vi "TicTacToe.vi"() -> ()   [LabVIEW 2017]
uses:
  Opponent.vi
panel:
  in  "Smart Computer":bool
  in  "New Game":bool
  in  "New Round":bool
  out "Score 2":i32
  out "Score 1":i32
  out "Status":string
  in  "Matrix":T1
  in  "Player 2":bool
  in  "Player 1":bool=TRUE
  # "Score"
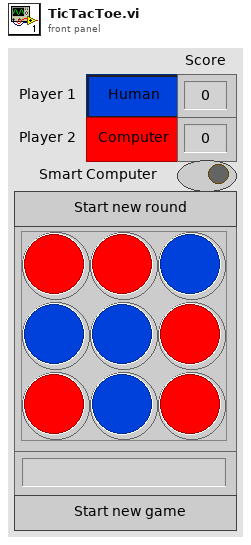
[diagram p1: front panel]
types:
  T1 = cluster{"0":bool, "1":bool, "2":bool, "3":bool, "4":bool, "5":bool, "6":bool, "7":bool, "8":bool}
  T2 = enum8{"Enabled", "Disabled", "Disabled and Grayed Out"}
  T3 = cluster{"Tokens":i32[][], "Score 1":i32, "Score 2":i32, "CurrentPlayer":i32, "FrontPanel":refnum<vi>, "StartPlayer":i32, "RoundRunning":bool}
  T4 = cluster{"Matrix[0]":bool, "Matrix[1]":bool, "Matrix[2]":bool, "Matrix[3]":bool, "Matrix[4]":bool, "Matrix[5]":bool, "Matrix[6]":bool, "Matrix[7]":bool, "Matrix[8]":bool}
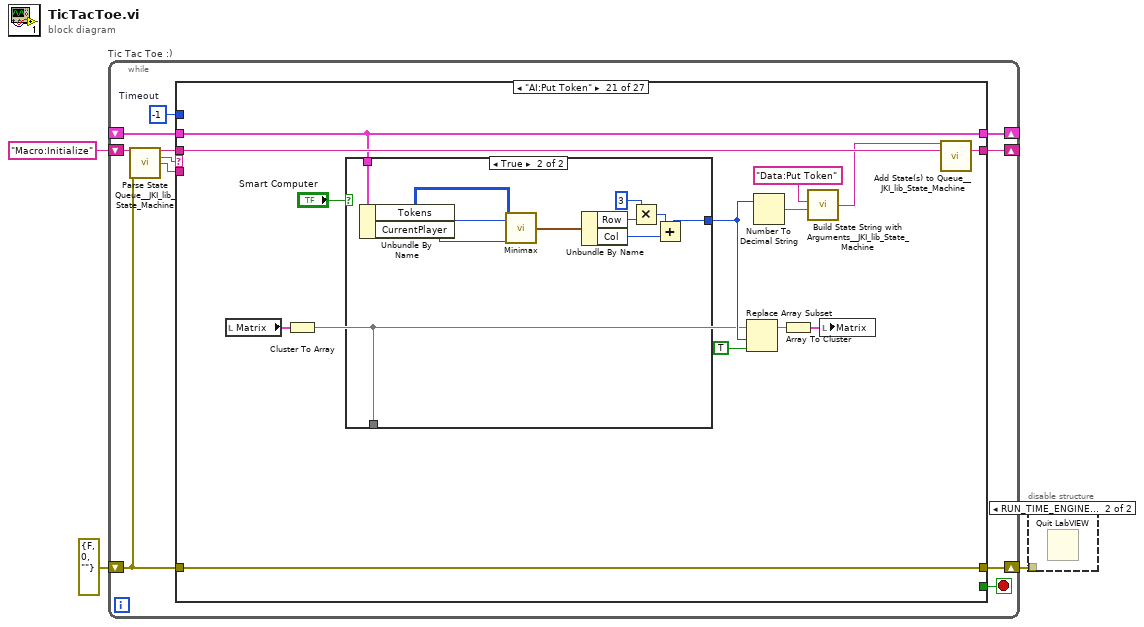
[diagram p0: block diagram]
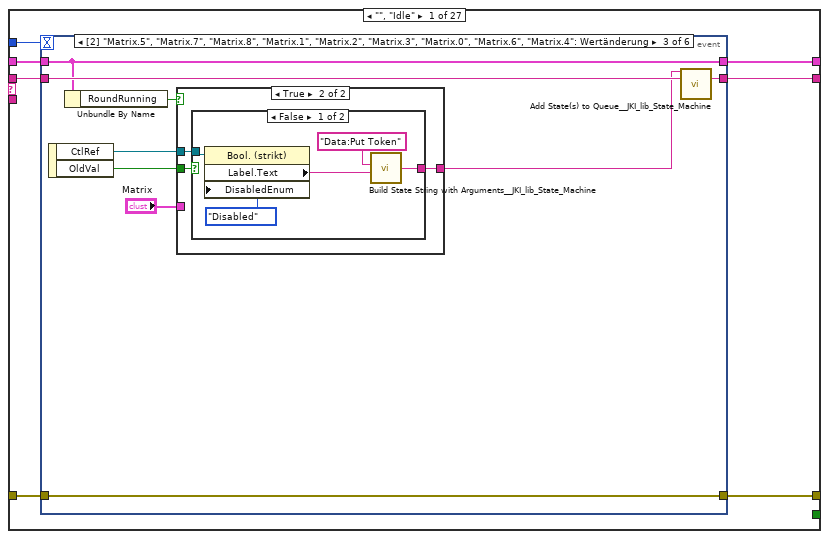
[diagram p3: hidden frame]
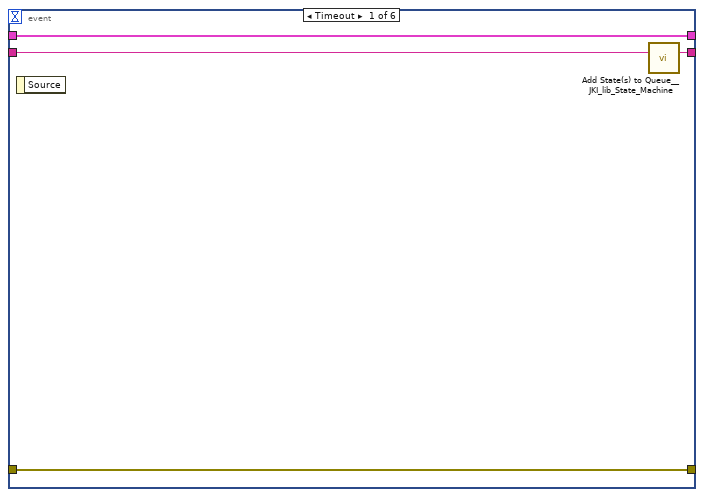
[diagram p4: hidden frame]
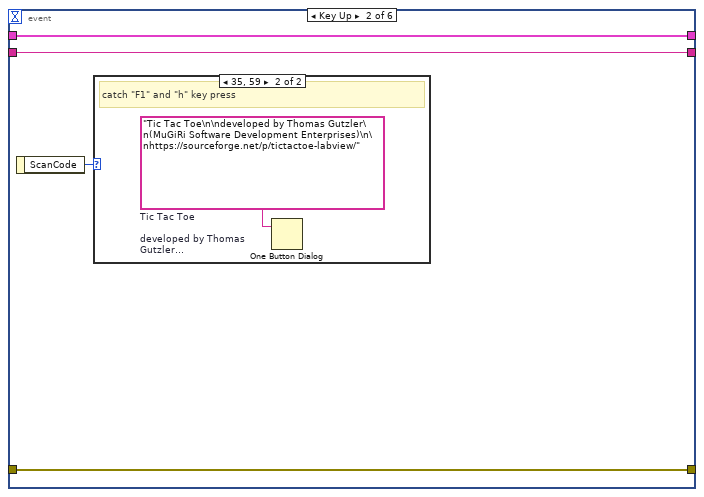
[diagram p5: hidden frame]
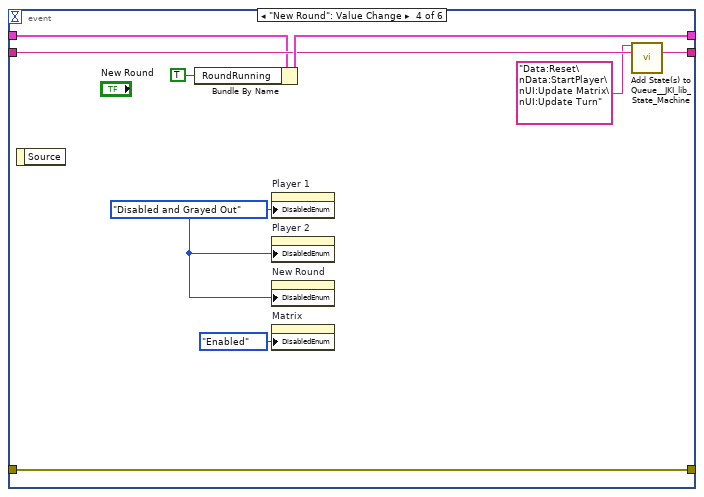
[diagram p9: hidden frame]
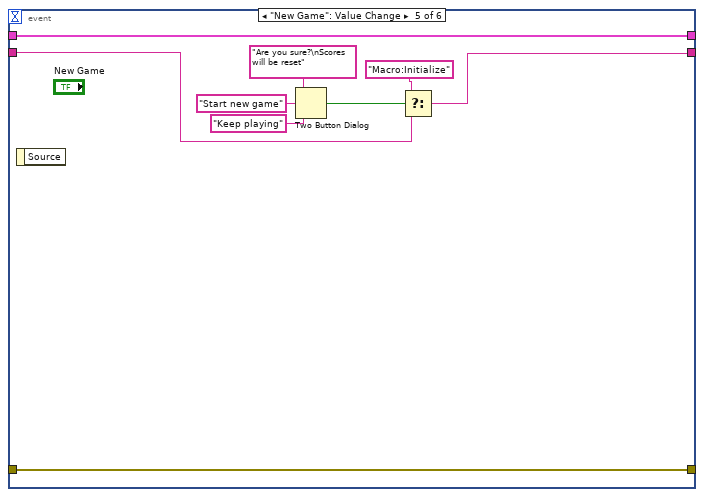
[diagram p10: hidden frame]
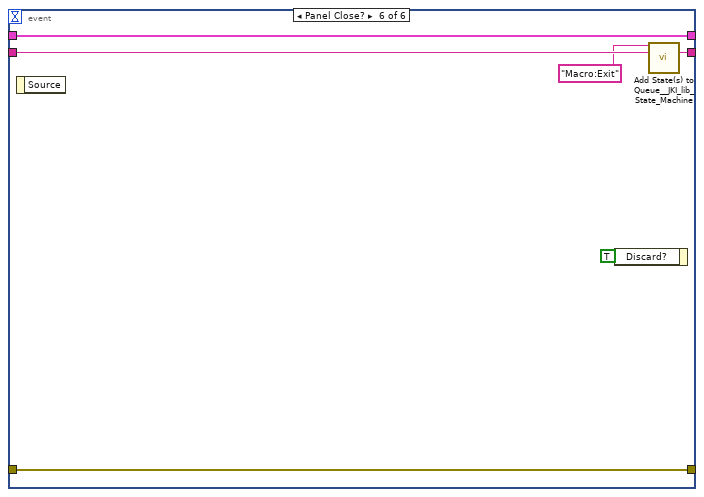
[diagram p11: hidden frame]
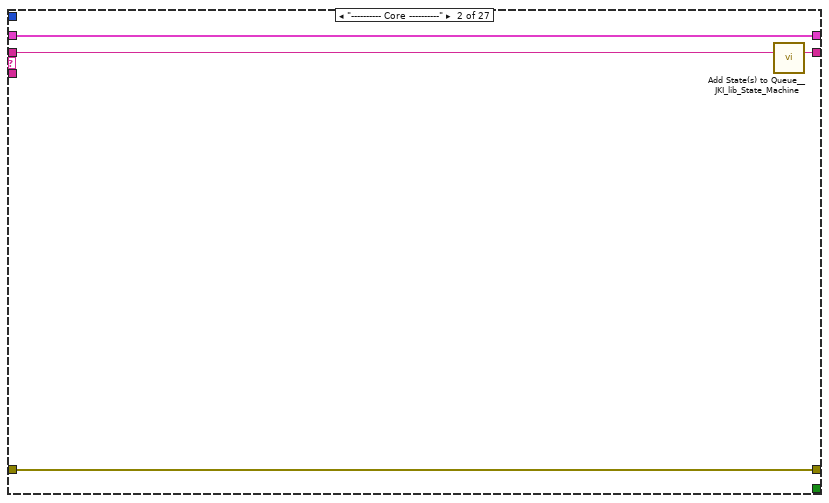
[diagram p12: hidden frame]
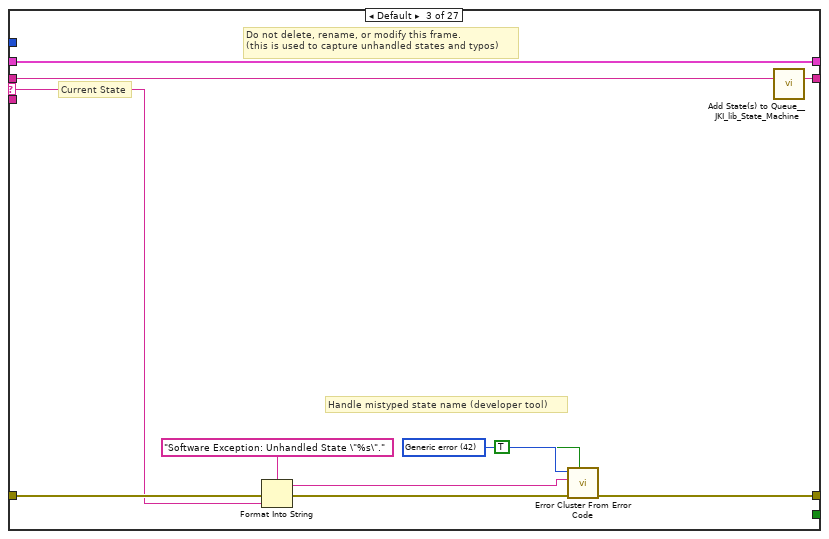
[diagram p13: hidden frame]
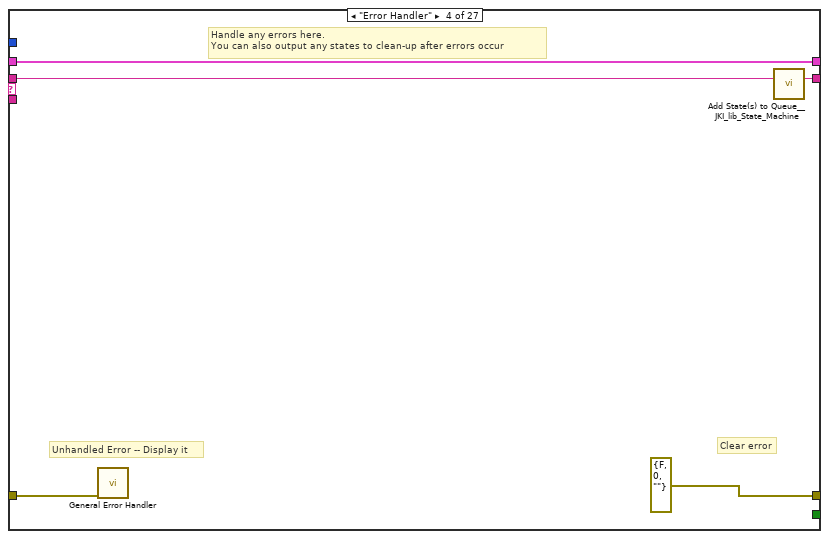
[diagram p14: hidden frame]
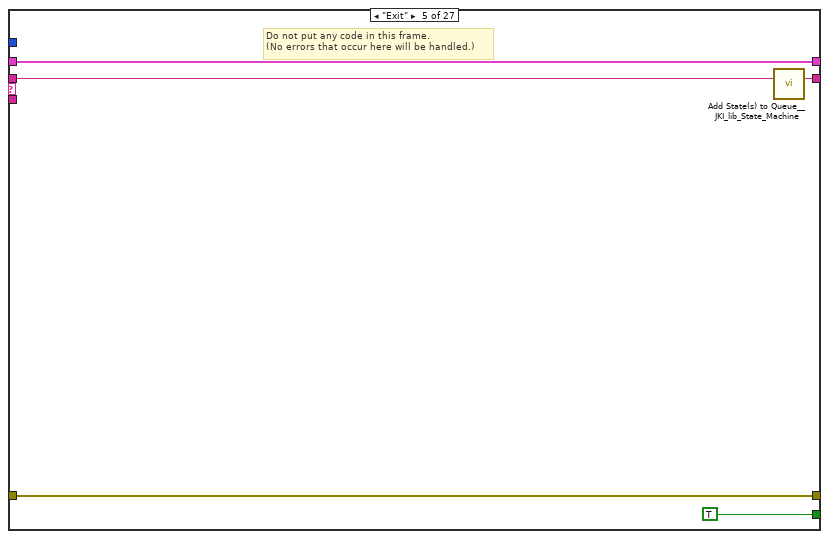
[diagram p15: hidden frame]
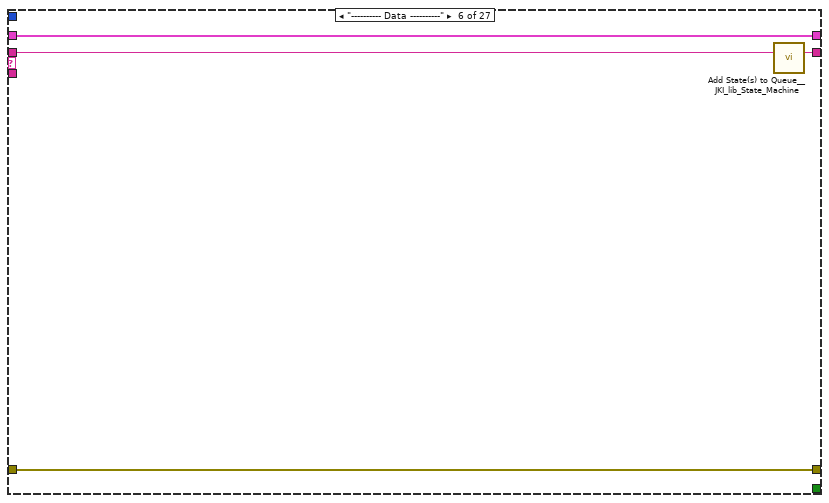
[diagram p16: hidden frame]
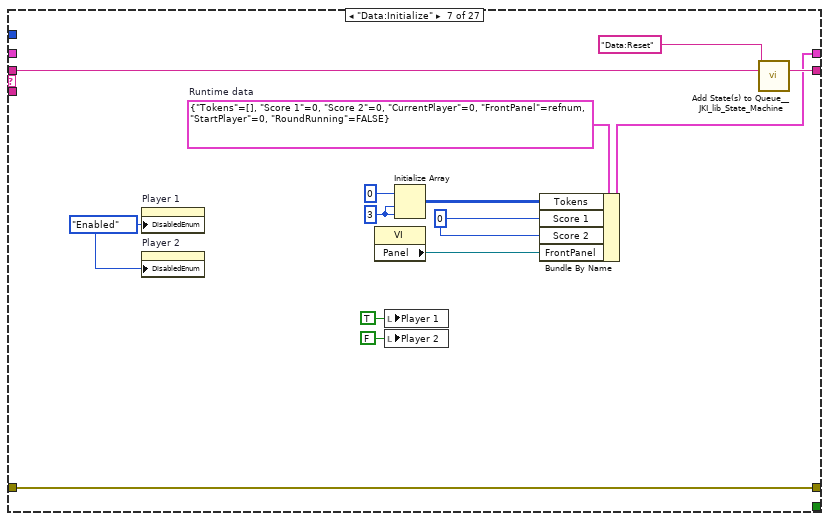
[diagram p17: hidden frame]
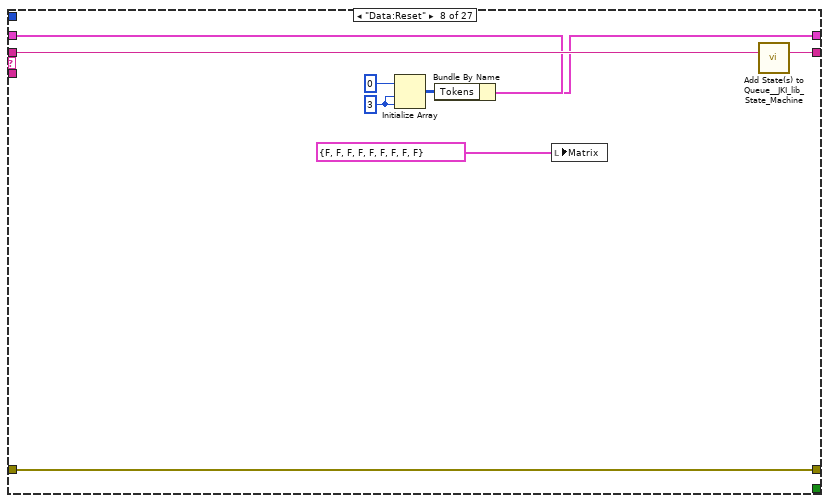
[diagram p18: hidden frame]
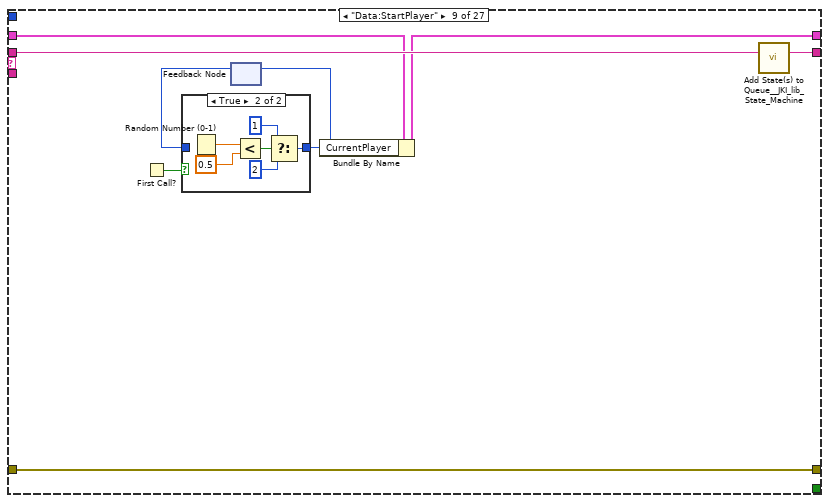
[diagram p19: hidden frame]
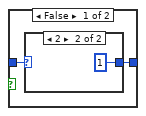
[diagram p20: hidden frame]
diagram:
  n1 = while "Tic Tac Toe :)" {
    shift-right: [w7] -> _
    shift-left: _ -> [w6]
    shift-right: [w10] -> w1
    shift-left: errorcluster {"status"=FALSE, "code"=0, "source"=""} ("error out") -> [w4]
    shift-right: [w9] -> _
    shift-left: "Macro:Initialize" -> [w11]
    stop <- w8 stop-if-true
    w5 = -1  # Timeout
    n2 = call <vilib>:"Parse State Queue__JKI_lib_State_Machine.vi"("State Queue"=w11, "Error In (no error)"=w4) -> ("Remaining States"=w13:string, "Current State"=w14:string, "Arguments"=w12:string)  [unwired: 11 in]
    n3 = case shown="\"AI:Put Token\"" w14 {
      selector: w14 -> [_ _ w76 _ _ _ _ _ _ _ _ _ _ _ _ _ _ _ _ _ _ _ _ _ _ _ _]
      tunnel: w13 -> [w21 w75 w80 w91 w96 w100 w114 w123 w131 w144 w180 w184 w193 w207 w230 w237 w242 w248 w252 w265 w279 w303 w308 w313 w317 _ _]
      tunnel: w12 -> [_ _ _ _ _ _ _ _ _ w162 w174 _ _ _ _ _ w239 _ _ _ _ _ _ _ _ w320 _]
      tunnel: w6 -> [w19 w72 w78 w88 w94 w97 _ w117 w128 w155 w177 w181 w191 w203 w227 w232 w240 w246 w249 w262 w269 w300 w305 w310 w314 w326 w342]
      tunnel: [w18 w73 w82 errorcluster {"status"=FALSE, "code"=0, "source"=""} ("error out") w93 w98 w112 w121 w129 w163 w178 w182 w190 w205 w228 w235 w238 w245 w250 w263 w277 w301 w306 w311 w315 w329 w348] -> w10
      tunnel: w4 -> [w17 w73 w81 w87 w93 w98 w112 w121 w129 w163 w178 w182 w190 w205 w228 w235 w238 w245 w250 w263 w277 w301 w306 w311 w315 w329 w348]
      tunnel: [w20 w74 w79 w90 w95 w99 w113 w122 w130 w145 w179 w183 w192 w206 w229 w236 w241 w247 w251 w264 w278 w302 w307 w312 w316 w330 "UI:Status >> Game Over"] -> w9
      tunnel: [_ _ _ _ TRUE _ _ _ _ _ _ _ _ _ _ _ _ _ _ _ _ _ _ _ _ _ _] -> w8
      tunnel: [w16 w72 w78 w88 w94 w97 w110 w116 w127 w160 w177 w181 w191 w203 w227 w232 w240 w246 w249 w262 w269 w300 w305 w310 w314 w325 w341] -> w7
      tunnel: w5 -> [w15 _ _ _ _ _ _ _ _ _ _ _ _ _ _ _ _ _ _ _ _ _ _ _ _ _ _]
      frame "", "Idle" {
        n4 = event shown="[2] \"Matrix.5\", \"Matrix.7\", \"Matrix.8\", \"Matrix.1\", \"Matrix.2\", \"Matrix.3\", \"Matrix.0\", \"Matrix.6\", \"Matrix.4\": Wertänderung" {
          selector: _ -> [_ _ _ _ _ _]
          dyn-events: _ -> [_ _ _ _ _ _]
          timeout: w15 -> [_ _ _ _ _ _]
          tunnel: w21 -> [w25 w27 w39 w53 w59 w71]
          tunnel: [w24 w27 w38 w52 w58 w70] -> w20
          tunnel: w19 -> [w22 w28 w31 w50 w65 w68]
          tunnel: [w23 w29 w37 w56 w57 w69] -> w18
          tunnel: w17 -> [w23 w29 w37 w56 w57 w69]
          tunnel: [w22 w28 w31 w55 w65 w68] -> w16
          event Timeout {
            n5 = event-data() -> ()  [unwired: 1 in, 1 out]
            n6 = call <vilib>:"Add State(s) to Queue__JKI_lib_State_Machine.vi"("State(s) in (\"\")"=w25) -> ("States Out"=w24:string)  [unwired: 14 in]
          }
          event Key Up {
            n7 = event-data() -> ("ScanCode"=w26:i16)  [unwired: 1 in]
            n8 = case shown="35, 59" w26 {
              frame 0, Default {
              }
              frame 35, 59 {
                w30 = "Tic Tac Toe\n\ndeveloped by Thomas Gutzler\n(MuGiRi Software Development Enterprises)\n\nhttps://sourceforge.net/p/tictactoe-labview/"  # Tic Tac Toe  developed by Thomas Gutzler (MuGiRi Software Development Enterprises)  https://sourceforge.net/p/tictactoe-labview/
                # "catch \"F1\" and \"h\" key press"
                n9 = One Button Dialog(message=w30) -> ()  [unwired: 1 in, 1 out]
              }
            }
          }
          event "Matrix.5", "Matrix.7", "Matrix.8", "Matrix.1", "Matrix.2", "Matrix.3", "Matrix.0", "Matrix.6", "Matrix.4": Value Change {
            n10 = event-data() -> ("CtlRef"=w36:refnum<vi>, "OldVal"=w34:bool)  [unwired: 1 in]
            n11 = Unbundle By Name(w31) -> ("RoundRunning"=w33:bool)
            n12 = case shown="True" w33 {
              tunnel: w36 -> [_ w42]
              tunnel: [_ w41] -> w35
              tunnel: w34 -> [_ w40]
              tunnel: "Matrix" -> [_ _]
              frame False {
              }
              frame True {
                n13 = case shown="False" w40 {
                  tunnel: w42 -> [w47 _]
                  tunnel: [w44 _] -> w41
                  frame False {
                    n14 = property class="Bool. (strikt)"(reference=w47, "DisabledEnum"=T2."Disabled" ("Disabled")) -> ("Label.Text"=w45:string)  [unwired: 1 in, 2 out]
                    n15 = call <vilib>:"Build State String with Arguments__JKI_lib_State_Machine.vi"("Arguments (\"\")"=w45, "State"="Data:Put Token") -> ("State with Arguments"=w44:string)  [unwired: 4 in]
                  }
                  frame True {
                  }
                }
              }
            }
            n16 = call <vilib>:"Add State(s) to Queue__JKI_lib_State_Machine.vi"("State(s) in Front (\"\")"=w35, "State(s) in (\"\")"=w39) -> ("States Out"=w38:string)  [unwired: 13 in]
          }
          event "New Round": Value Change {
            w51 = T2."Disabled and Grayed Out" ("Disabled")
            n17 = event-data() -> ()  [unwired: 1 in, 1 out]
            n18 = Bundle By Name(cluster=w50, "RoundRunning"=TRUE ("GameRunning")) -> (w55:T3)
            n19 = property on="Player 1" class="Bool. (strikt)"("DisabledEnum"=w51) -> ()  [unwired: 2 in, 2 out]
            n20 = property on="Player 2" class="Bool. (strikt)"("DisabledEnum"=w51) -> ()  [unwired: 2 in, 2 out]
            n21 = property on="New Round" class="Bool. (strikt)"("DisabledEnum"=w51) -> ()  [unwired: 2 in, 2 out]
            n22 = property on="Matrix" class="Cluster (strikt)"("DisabledEnum"=T2."Enabled" ("Disabled")) -> ()  [unwired: 2 in, 2 out]
            n23 = call <vilib>:"Add State(s) to Queue__JKI_lib_State_Machine.vi"("State(s) in Front (\"\")"="Data:Reset\nData:StartPlayer\nUI:Update Matrix\nUI:Update Turn", "State(s) in (\"\")"=w53) -> ("States Out"=w52:string)  [unwired: 13 in]
          }
          event "New Game": Value Change {
            n24 = event-data() -> ()  [unwired: 1 in, 1 out]
            n25 = Two Button Dialog(message="Are you sure?\nScores will be reset", 1:"Keep playing", 2:"Start new game" ("T button name (\"OK\")")) -> (T button?=w61:bool)
            n26 = Select(t="Macro:Initialize", s=w61, f=w59) -> (s? t:f=w58:string)
          }
          event Panel Close? {
            n27 = event-data() -> ()  [unwired: 1 in, 1 out]
            n28 = event-data("Discard?"=TRUE) -> ()  [unwired: 1 in, 1 out]
            n29 = call <vilib>:"Add State(s) to Queue__JKI_lib_State_Machine.vi"("State(s) in Front (\"\")"="Macro:Exit", "State(s) in (\"\")"=w71) -> ("States Out"=w70:string)  [unwired: 13 in]
          }
        }
      }
      frame "---------- Core ----------" {
        n30 = call <vilib>:"Add State(s) to Queue__JKI_lib_State_Machine.vi"("State(s) in (\"\")"=w75) -> ("States Out"=w74:string)  [unwired: 14 in]
      }
      frame Default {
        w85 = 42 items=["No error", "Argument error", "Memory is full", "Out of zone", "End of file", "File already open", "Generic file I/O error", "File not found", "File permission error", "Disk is full", "Duplicate path", "Too many files open", "System feature not enabled", "Resource file not found", "Cannot add resource", "Resource not found", "Image not found", "Image memory error", "Pen does not exist", "Config type invalid", "Config token not found", "Config parse error", "Config memory error", "Bad external code format", "Bad external code offset", "External code not present", "Null window", "Destroy window error", "Null menu", "Print aborted", "Bad print record", "Print driver error", "Windows error during printing", "Memory error during printing", "Print dialog error", "Generic print error", "Invalid device refnum", "Device not found", "Device parameter error", "Device unit error", "Cannot open device", "Device call aborted", "Generic error", "Cancelled by user", "Object ID too low", "Object ID too high", "Object not in heap", "Unknown heap", "Unknown object (invalid DefProc)", "Unknown object (DefProc not in table)", "Message out of range", "Invalid (null) method", "Unknown message", "Manager call not supported", "Bad address", "Network operation in progress", "Network operation timed out", "Connection is busy", "Network attribute not supported", "Network error", "Address in use", "System out of memory", "Connection aborted", "Connection refused", "Not connected", "Already connected", "Connection closed", "Initialization error (interapplication manager)", "Bad occurrence", "Wait on unbound occurrence handler", "Occurrence queue overflow", "Datalog type conflict", "Unused", "Unrecognized type (interapplication manager)", "Memory corrupt", "Failed to make temporary DLL", "Old CIN version", "Drag socket not found", "Failed to load drop-object", "Failed to register OLE object", "Failed to release OLE object", "Format specifier type mismatch", "Unknown format specifier", "Too few format specifiers", "Too many format specifiers", "Scan failed", "Newer CIN version", "Error converting to variant", "Runtime menu error", "Password tampered", "Variant attribute not found", "Incompatible variant data type", "Event data is not available", "Event Store is not present", "Occurrence is not found", "Event Queue is not created", "Event info is not available", "Refnum passed is NULL", "Error retrieving Class GUID", "Error retrieving CoClass GUID", "Error retrieving TypeLib GUID.", "Bad built application magic bytes.", "Specific driver is different from the specific driver associated with the Logical Name.", "There is no session opened to the class driver.", "Max Error", "MAX - Error with config objects", "MAX - Error loading configuration", "MAX - Group not supported"]
        # "Current State"
        # "Do not delete, rename, or modify this frame.\n(this is used to capture unhandled states and typos)"
        # "Handle mistyped state name (developer tool)"
        n31 = Format Into String(format string="Software Exception: Unhandled State \"%s\"." ("message"), error in=w81, w76) -> (resulting string=w84:string, error out=w83:errorcluster)  [unwired: 1 in]
        n32 = call <vilib>:"Error Cluster From Error Code.vi"("show call chain? (False)"=TRUE, "error in (no error)"=w83, "error message (\"\")"=w84, "error code (0)"=w85) -> ("error out"=w82:errorcluster)  [unwired: 5 in]
        n33 = call <vilib>:"Add State(s) to Queue__JKI_lib_State_Machine.vi"("State(s) in (\"\")"=w80) -> ("States Out"=w79:string)  [unwired: 14 in]
      }
      frame "Error Handler" {
        # "Unhandled Error -- Display it"
        # "Handle any errors here.\nYou can also output any states to clean-up after errors occur"
        # "Clear error"
        n34 = call <vilib>:"General Error Handler.vi"("error in (no error)"=w87) -> ()  [unwired: 10 in, 5 out]
        n35 = call <vilib>:"Add State(s) to Queue__JKI_lib_State_Machine.vi"("State(s) in (\"\")"=w91) -> ("States Out"=w90:string)  [unwired: 14 in]
      }
      frame "Exit" {
        # "Do not put any code in this frame.\n(No errors that occur here will be handled.)"
        n36 = call <vilib>:"Add State(s) to Queue__JKI_lib_State_Machine.vi"("State(s) in (\"\")"=w96) -> ("States Out"=w95:string)  [unwired: 14 in]
      }
      frame "---------- Data ----------" {
        n37 = call <vilib>:"Add State(s) to Queue__JKI_lib_State_Machine.vi"("State(s) in (\"\")"=w100) -> ("States Out"=w99:string)  [unwired: 14 in]
      }
      frame "Data:Initialize" {
        w102 = T2."Enabled" ("Disabled")
        w105 = 3 ("Score 1")
        w107 = 0 ("Score 1")
        w111 = T3 {"Tokens"=[], "Score 1"=0, "Score 2"=0, "CurrentPlayer"=0, "FrontPanel"=refnum, "StartPlayer"=0, "RoundRunning"=FALSE}  # Runtime data
        n38 = property on="Player 1" class="Bool. (strikt)"("DisabledEnum"=w102) -> ()  [unwired: 2 in, 2 out]
        n39 = property on="Player 2" class="Bool. (strikt)"("DisabledEnum"=w102) -> ()  [unwired: 2 in, 2 out]
        n40 = property class="VI"() -> ("Panel"=w106:refnum<vi>)  [unwired: 2 in, 2 out]
        n41 = local write "Player 1"(TRUE ("Player 1")) -> ()
        n42 = local write "Player 2"(FALSE ("Player 2")) -> ()
        n43 = Initialize Array(0 ("Score 1"), w105, w105) -> (w108:i32[][])
        n44 = Bundle By Name(cluster=w111, "Tokens"=w108, "Score 1"=w107, "Score 2"=w107, "FrontPanel"=w106) -> (w110:T3)
        n45 = call <vilib>:"Add State(s) to Queue__JKI_lib_State_Machine.vi"("State(s) in Front (\"\")"="Data:Reset", "State(s) in (\"\")"=w114) -> ("States Out"=w113:string)  [unwired: 13 in]
      }
      frame "Data:Reset" {
        w118 = 3 ("Score 1")
        n46 = Initialize Array(0 ("Score 1"), w118, w118) -> (w119:i32[][])
        n47 = Bundle By Name(cluster=w117, "Tokens"=w119) -> (w116:T3)
        n48 = local write "Matrix"(T1 {"0"=FALSE, "1"=FALSE, "2"=FALSE, "3"=FALSE, "4"=FALSE, "5"=FALSE, "6"=FALSE, "7"=FALSE, "8"=FALSE} ("Matrix")) -> ()
        n49 = call <vilib>:"Add State(s) to Queue__JKI_lib_State_Machine.vi"("State(s) in (\"\")"=w123) -> ("States Out"=w122:string)  [unwired: 14 in]
      }
      frame "Data:StartPlayer" {
        n50 = First Call?() -> (First Call?: T/F=w126:bool)
        n51 = feedback #1() -> (w124:i32)  [unwired: 1 in]
        n52 = case shown="True" w126 {
          tunnel: [w132 w136] -> w125
          tunnel: w124 -> [w133 _]
          frame False {
            n53 = case shown="2" w133 {
              tunnel: [2 1] -> w132
              frame Default {
              }
              frame 2 {
              }
            }
          }
          frame True {
            n54 = Random Number (0-1)() -> (number: 0 to 1=w141:dbl)
            n55 = Less?(x=w141, y=0.5 ("x")) -> (x < y?=w139:bool)
            n56 = Select(t=1 ("Score 2"), s=w139, f=2 ("Score 2")) -> (s? t:f=w136:i32)
          }
        }
        n57 = feedback-in #1(w125) -> ()
        n58 = Bundle By Name(cluster=w128, "CurrentPlayer"=w125) -> (w127:T3)
        n59 = call <vilib>:"Add State(s) to Queue__JKI_lib_State_Machine.vi"("State(s) in (\"\")"=w131) -> ("States Out"=w130:string)  [unwired: 14 in]
      }
      frame "Data:Put Token" {
        w153 = 3 ("dimension size")
        n60 = Decimal String To Number(string=w162) -> (number=w161:i32)  [unwired: 2 in, 1 out]
        n61 = Unbundle By Name(w155) -> ("CurrentPlayer"=w149:i32)
        n62 = Unbundle By Name(w155) -> ("Tokens"=w157:i32[][])
        n63 = Reshape Array(w157, 9 ("dimension size")) -> (w156:i32[])
        n64 = Replace Array Subset(array=w156, new element=w149, index=w161) -> (w154:i32[])
        n65 = case shown="Standard" w149 {
          tunnel: [1 ("CurrentPlayer") 2 ("CurrentPlayer")] -> w151
          frame Default {
          }
          frame 1 {
          }
        }
        n66 = Number To Decimal String(number=w149) -> (decimal integer string=w148:string)  [unwired: 1 in]
        n67 = Reshape Array(w154, w153, w153) -> (w152:i32[][])
        n68 = Bundle By Name(cluster=w155, "Tokens"=w152, "CurrentPlayer"=w151) -> (w160:T3)
        n69 = call <vilib>:"Build State String with Arguments__JKI_lib_State_Machine.vi"("Arguments (\"\")"=w148, "State"="Data:Check Win") -> ("State with Arguments"=w147:string)  [unwired: 4 in]
        n70 = call <vilib>:"Add State(s) to Queue__JKI_lib_State_Machine.vi"("State(s) in Front (\"\")"="UI:Update Turn", "State(s) in (\"\")"=w144) -> ("States Out"=w143:string)  [unwired: 13 in]
        n71 = call <vilib>:"Add State(s) to Queue__JKI_lib_State_Machine.vi"("State(s) in Front (\"\")"=w147, "State(s) in (\"\")"=w143) -> ("States Out"=w146:string)  [unwired: 13 in]
        n72 = call <vilib>:"Add State(s) to Queue__JKI_lib_State_Machine.vi"("State(s) in Front (\"\")"="UI:Update Matrix", "State(s) in (\"\")"=w146) -> ("States Out"=w145:string)  [unwired: 13 in]
      }
      frame "Data:Check Win" {
        n73 = Unbundle By Name(w177) -> ("Tokens"=w172:i32[][])
        n74 = Decimal String To Number(string=w174) -> (number=w171:i32)  [unwired: 2 in, 1 out]
        n75 = call "Score.vi"("Turn Taking Player"=w171, "Game"=w172) -> ("Game over"=w169:bool, "Win"=w170:bool)  [unwired: 7 in, 1 out]
        n76 = Select(t="Game:Over", s=w169, f="") -> (s? t:f=w166:string)
        n77 = call <vilib>:"Build State String with Arguments__JKI_lib_State_Machine.vi"("Arguments (\"\")"=w174, "State"="Game:Winner") -> ("State with Arguments"=w173:string)  [unwired: 4 in]
        n78 = Select(t=w173, s=w170, f=w166) -> (s? t:f=w176:string)
        n79 = call <vilib>:"Add State(s) to Queue__JKI_lib_State_Machine.vi"("State(s) in Front (\"\")"=w176, "State(s) in (\"\")"=w180) -> ("States Out"=w179:string)  [unwired: 13 in]
      }
      frame "---------- UI ----------" {
        n80 = call <vilib>:"Add State(s) to Queue__JKI_lib_State_Machine.vi"("State(s) in (\"\")"=w184) -> ("States Out"=w183:string)  [unwired: 14 in]
      }
      frame "UI:Initialize" {
        # "Initialize the User Interface, here.\n(this is called automatically, by the Macro: Init)"
        n81 = property on="New Round" class="Bool. (strikt)"("DisabledEnum"=T2."Enabled" ("Disabled")) -> ()  [unwired: 2 in, 2 out]
        n82 = property on="Matrix" class="Cluster (strikt)"("DisabledEnum"=T2."Disabled" ("Disabled")) -> ()  [unwired: 2 in, 2 out]
        n83 = local write "New Round"(FALSE ("Start")) -> ()
        n84 = local write "Matrix"(T1 {"0"=FALSE, "1"=FALSE, "2"=FALSE, "3"=FALSE, "4"=FALSE, "5"=FALSE, "6"=FALSE, "7"=FALSE, "8"=FALSE} ("Matrix")) -> ()
        n85 = call <vilib>:"Add State(s) to Queue__JKI_lib_State_Machine.vi"("State(s) in Front (\"\")"="UI:Status\nUI:Update Score\nUI:Update Matrix", "State(s) in (\"\")"=w193) -> ("States Out"=w192:string)  [unwired: 13 in]
      }
      frame "UI:Update Matrix" {
        n86 = Unbundle By Name(w203) -> ("FrontPanel"=w202:refnum<vi>)
        n87 = property class="Pnl"(reference=w202, "DeferPanUpdts"=TRUE ("Defer Panel Updates")) -> (reference out=w199:refnum<vi>, error out=w200:errorcluster)  [unwired: 1 in]
        n88 = property on="Matrix" class="Cluster (strikt)"(error in=w200) -> ("Controls[]"=w204:refnum<vi>[])  [unwired: 1 in, 2 out]
        n89 = Unbundle By Name(w203) -> ("Tokens"=w196:i32[][])
        n90 = Reshape Array(w196, 9 ("dimension size")) -> (w194:i32[])
        n91 = for {
          tunnel: w204 -> [w218] mode=indexing
          tunnel: w194 -> [w212]
          tunnel: [w210] -> w198
          w216 = refnum<vi> refnum  # Boolesch
          n92 = To More Specific Class(target class=w216, reference=w218) -> (specific class reference=w217:refnum<vi>)  [unwired: 1 in, 1 out]
          n93 = property class="Bool."(reference=w217) -> (reference out=w215:refnum<vi>, "Label.Text"=w214:string)  [unwired: 1 in, 1 out]
          n94 = Decimal String To Number(string=w214) -> (number=w213:i32)  [unwired: 2 in, 1 out]
          n95 = Index Array(array=w212, index=w213) -> (element=w209:i32)
          n96 = case shown="Standard" w209 {
            tunnel: [cluster{u32, u32}[] [{13816530, 13816530}, {13816530, 13816530}] ("Colors [4]") cluster{u32, u32}[] [{16860, 16860}, {16860, 16860}] ("Colors [4]") cluster{u32, u32}[] [{16711680, 16711680}, {16711680, 16711680}] ("Colors [4]")] -> w211
            tunnel: [T2."Enabled" ("Disabled") T2."Disabled" ("Disabled") T2."Disabled" ("Disabled")] -> w208
            frame Default {
            }
            frame 1 {
            }
            frame 2 {
            }
          }
          n97 = property class="Bool."(reference=w215, "Colors [4]"=w211, "DisabledEnum"=w208) -> (error out=w210:errorcluster)  [unwired: 1 in, 1 out]
        }
        n98 = property class="Pnl"(reference=w199, error in=w198, "DeferPanUpdts"=FALSE ("Defer Panel Updates")) -> ()  [unwired: 2 out]
        n99 = call <vilib>:"Add State(s) to Queue__JKI_lib_State_Machine.vi"("State(s) in (\"\")"=w207) -> ("States Out"=w206:string)  [unwired: 14 in]
      }
      frame "UI:Update Score" {
        n100 = Unbundle By Name(w227) -> ("Score 1"=→"Score 1":i32, "Score 2"=→"Score 2":i32)
        n101 = call <vilib>:"Add State(s) to Queue__JKI_lib_State_Machine.vi"("State(s) in (\"\")"=w230) -> ("States Out"=w229:string)  [unwired: 14 in]
      }
      frame "UI:Update Turn" {
        n102 = Unbundle By Name(w232) -> ("CurrentPlayer"=w233:i32)
        n103 = Format Into String(format string="UI:Status >> Player %d's turn\nAI:Check Turn", w233) -> (resulting string=w231:string)  [unwired: 2 in, 1 out]
        n104 = call <vilib>:"Add State(s) to Queue__JKI_lib_State_Machine.vi"("State(s) in Front (\"\")"=w231, "State(s) in (\"\")"=w237) -> ("States Out"=w236:string)  [unwired: 13 in]
      }
      frame "UI:Status" {
        n105 = call <vilib>:"Add State(s) to Queue__JKI_lib_State_Machine.vi"("State(s) in (\"\")"=w242) -> ("States Out"=w241:string)  [unwired: 14 in]
        "Status" <- w239
      }
      frame "UI:Cleanup" {
        w244 = T2."Enabled" ("Disabled")
        n106 = local write "New Round"(FALSE ("Start")) -> ()
        n107 = property on="Player 1" class="Bool. (strikt)"("DisabledEnum"=w244) -> ()  [unwired: 2 in, 2 out]
        n108 = property on="Player 2" class="Bool. (strikt)"("DisabledEnum"=w244) -> ()  [unwired: 2 in, 2 out]
        n109 = call <vilib>:"Add State(s) to Queue__JKI_lib_State_Machine.vi"("State(s) in (\"\")"=w248) -> ("States Out"=w247:string)  [unwired: 14 in]
      }
      frame "---------- AI ----------" {
        n110 = call <vilib>:"Add State(s) to Queue__JKI_lib_State_Machine.vi"("State(s) in (\"\")"=w252) -> ("States Out"=w251:string)  [unwired: 14 in]
      }
      frame "AI:Check Turn" {
        n111 = Unbundle By Name(w262) -> ("CurrentPlayer"=w258:i32)
        n112 = Decrement(x=w258) -> (x-1=w257:i32)
        n113 = Build Array("Player 1", "Player 2") -> (w259:bool[])
        n114 = Index Array(array=w259, index=w257) -> (element=w256:bool)
        n115 = Select(t="", s=w256, f="AI:Put Token") -> (s? t:f=w255:string)
        n116 = call <vilib>:"Add State(s) to Queue__JKI_lib_State_Machine.vi"("State(s) in Front (\"\")"=w255, "State(s) in (\"\")"=w265) -> ("States Out"=w264:string)  [unwired: 13 in]
      }
      frame "AI:Put Token" {
        n117 = local read "Matrix"() -> (w276:T1)
        n118 = Cluster To Array(cluster=w276) -> (array=w266:bool[])
        n119 = case shown="True" "Smart Computer" {
          tunnel: w269 -> [_ w299]
          tunnel: [w281 w291] -> w268
          tunnel: w266 -> [w280 _]
          frame False {
            n120 = Not(x=w280) -> (.not. x?=w283:bool[])
            n121 = Boolean To (0,1)(Boolean=w283) -> (0, 1=w282:i16[])
            n122 = for {
              tunnel: [w290] -> w284 mode=indexing if=w289
              tunnel: w283 -> [w289] mode=indexing
              i -> [w290]
            }
            n123 = Add Array Elements(numeric array=w282) -> (sum=w286:i16)
            n124 = Random Number (0-1)() -> (number: 0 to 1=w285:dbl)
            n125 = Decrement(x=w286) -> (x-1=w287:i16)
            n126 = Multiply(x=w287, y=w285) -> (x*y=w288:dbl)
            n127 = Index Array(array=w284, index=w288) -> (element=w281:i32)
          }
          frame True {
            n128 = Unbundle By Name(w299) -> ("Tokens"=w298:i32[][], "CurrentPlayer"=w297:i32)
            n129 = call "Minimax.vi"("Game"=w298, "Active Turn"=w297, "Turn Taking Player"=w297) -> ("Next Move"=w296:cluster{"Row":i32, "Col":i32})  [unwired: 13 in, 3 out]
            n130 = Unbundle By Name(w296) -> ("Row"=w295:i32, "Col"=w292:i32)
            n131 = Multiply(x=3, y=w295) -> (x*y=w293:i32)
            n132 = Add(x=w293, y=w292) -> (x+y=w291:i32)
          }
        }
        n133 = Replace Array Subset(array=w266, new element=TRUE ("new element/subarray"), index=w268) -> (w271:bool[])
        n134 = Number To Decimal String(number=w268) -> (decimal integer string=w274:string)  [unwired: 1 in]
        n135 = Array To Cluster(array=w271) -> (cluster=w270:T4)
        n136 = call <vilib>:"Build State String with Arguments__JKI_lib_State_Machine.vi"("Arguments (\"\")"=w274, "State"="Data:Put Token") -> ("State with Arguments"=w273:string)  [unwired: 4 in]
        n137 = local write "Matrix"(w270) -> ()
        n138 = call <vilib>:"Add State(s) to Queue__JKI_lib_State_Machine.vi"("State(s) in Front (\"\")"=w273, "State(s) in (\"\")"=w279) -> ("States Out"=w278:string)  [unwired: 13 in]
      }
      frame "---------- Macro ----------" {
        n139 = call <vilib>:"Add State(s) to Queue__JKI_lib_State_Machine.vi"("State(s) in (\"\")"=w303) -> ("States Out"=w302:string)  [unwired: 14 in]
      }
      frame "Macro:Initialize" {
        # "Initialization Macro\n(This is called when the VI starts and a new game is started)"
        n140 = call <vilib>:"Add State(s) to Queue__JKI_lib_State_Machine.vi"("State(s) in Front (\"\")"="Data:Initialize\nUI:Initialize", "State(s) in (\"\")"=w308) -> ("States Out"=w307:string)  [unwired: 13 in]
      }
      frame "Macro:Exit" {
        # "Exit Macro\n(This is called once, when the VI exits)"
        n141 = call <vilib>:"Add State(s) to Queue__JKI_lib_State_Machine.vi"("State(s) in Front (\"\")"="UI:Cleanup\nExit", "State(s) in (\"\")"=w313) -> ("States Out"=w312:string)  [unwired: 13 in]
      }
      frame "---------- Game ----------" {
        n142 = call <vilib>:"Add State(s) to Queue__JKI_lib_State_Machine.vi"("State(s) in (\"\")"=w317) -> ("States Out"=w316:string)  [unwired: 14 in]
      }
      frame "Game:Winner" {
        n143 = Decimal String To Number(string=w320) -> (number=w319:i32)  [unwired: 2 in, 1 out]
        n144 = case shown="2" w319 {
          tunnel: w326 -> [w335 w340]
          tunnel: w326 -> [w334 w339]
          tunnel: [w333 w338] -> w327
          frame Default {
            n145 = Unbundle By Name(w335) -> ("Score 1"=w332:i32)
            n146 = Increment(x=w332) -> (x+1=w331:i32)
            n147 = Bundle By Name(cluster=w334, "Score 1"=w331) -> (w333:T3)
          }
          frame 2 {
            n148 = Unbundle By Name(w340) -> ("Score 2"=w337:i32)
            n149 = Increment(x=w337) -> (x+1=w336:i32)
            n150 = Bundle By Name(cluster=w339, "Score 2"=w336) -> (w338:T3)
          }
        }
        n151 = property on="New Round" class="Bool. (strikt)"("DisabledEnum"=T2."Enabled" ("Disabled"), "Value"=FALSE ("Start")) -> ()  [unwired: 2 in, 2 out]
        n152 = property on="Matrix" class="Cluster (strikt)"("DisabledEnum"=T2."Disabled" ("Disabled")) -> ()  [unwired: 2 in, 2 out]
        n153 = Format Into String(format string="UI:Update Score\nUI:Status >> Player %d has won", w319) -> (resulting string=w322:string)  [unwired: 2 in, 1 out]
        n154 = Bundle By Name(cluster=w327, "RoundRunning"=FALSE) -> (w325:T3)
        n155 = call <vilib>:"Add State(s) to Queue__JKI_lib_State_Machine.vi"("State(s) in Front (\"\")"=w322) -> ("States Out"=w330:string)  [unwired: 14 in]
      }
      frame "Game:Over" {
        n156 = property on="New Round" class="Bool. (strikt)"("DisabledEnum"=T2."Enabled" ("Disabled"), "Value"=FALSE ("Start")) -> ()  [unwired: 2 in, 2 out]
        n157 = property on="Matrix" class="Cluster (strikt)"("DisabledEnum"=T2."Disabled" ("Disabled")) -> ()  [unwired: 2 in, 2 out]
        n158 = Bundle By Name(cluster=w342, "RoundRunning"=FALSE) -> (w341:T3)
      }
    }
  }
  n159 = disable-structure shown="RUN_TIME_ENGINE==True" {
    disable-tunnel: w1 -> [_ _]
    frame condition #0 (active) {
    }
    frame condition #1 {
      n160 = Quit LabVIEW() -> ()  [unwired: 1 in]
    }
  }
